vi "Read Topic Filter.vi"(8 "error in (no error)":errorcluster, 11 "Subscription in":refnum<class "Subscription.lvclass">) -> (0 "error out":errorcluster, 2 "Topic Filter":string, 3 "Subscription out":refnum<class "Subscription.lvclass">)   [LabVIEW 2013, in "MQTT Server.lvlib" / "Subscription.lvclass"]
uses:
  Subscription.lvclass
  Subscription.lvclass/Subscription.ctl
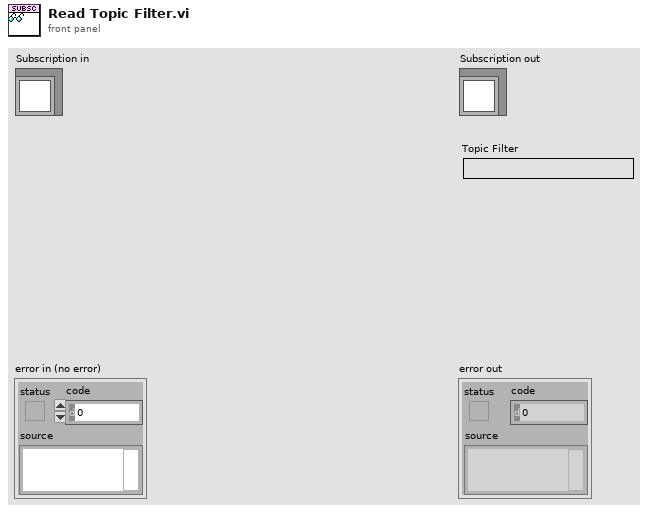
[diagram p1: front panel]
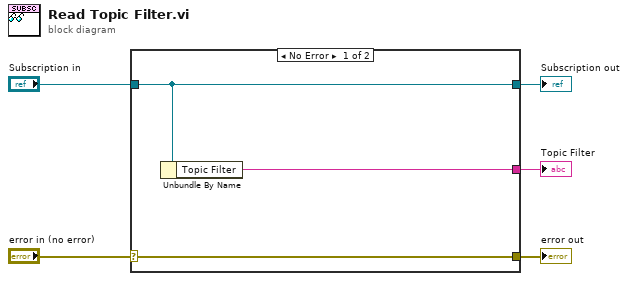
[diagram p0: block diagram]
diagram:
  n1 = case shown="No Error" "error in (no error)" {
    selector: "error in (no error)" -> [w8 w9]
    tunnel: [w8 w9] -> w4
    tunnel: [w7 w10] -> w2
    tunnel: "Subscription in" -> [w7 w10]
    tunnel: [w6 _] -> w1
    frame No Error {
      n2 = Unbundle By Name(w7) -> ("Topic Filter"=w6:string)
    }
    frame Error {
    }
  }
  "error out" <- w4
  "Subscription out" <- w2
  "Topic Filter" <- w1
